vi "Save Data To File.vi"(0 "VISA resource name":refnum<visa-resource-name>, 1 "Memory Waveform Source (0: Channel 1)":i32(ring) items=["Channel 1", "Channel 2", "Channel 3", "Channel 4", "Math", "Memory Waveform 1", "Memory Waveform 2"], 2 "Internal Location (0)":dbl, 5 "File Type (0: Agilent Logic Binary)":i32(ring) items=["Agilent Logic Binary", "ASCII XY ", "CSV", "Binary", "Reference Waveform", "Setup", "Lister", "Masker", "Arbitrary", "Power"], 7 "Waveform Length (2000 points)":i32=2000, 9 "Segment Select (0: All)":i32(ring) items=["All", "Current"], 11 "error in (no error)":errorcluster, 12 "File Name":string, 13 "Enable Max Waveform Length (F: Disable)":bool) -> (4 "VISA resource name out":refnum<visa-resource-name>, 15 "error out":errorcluster)   [LabVIEW 2023, in "Keysight-DSQx3014T.lvlib"]
doc: "Configure the save waveform to file operation."
uses:
  Keysight-DSQx3014T.lvlib
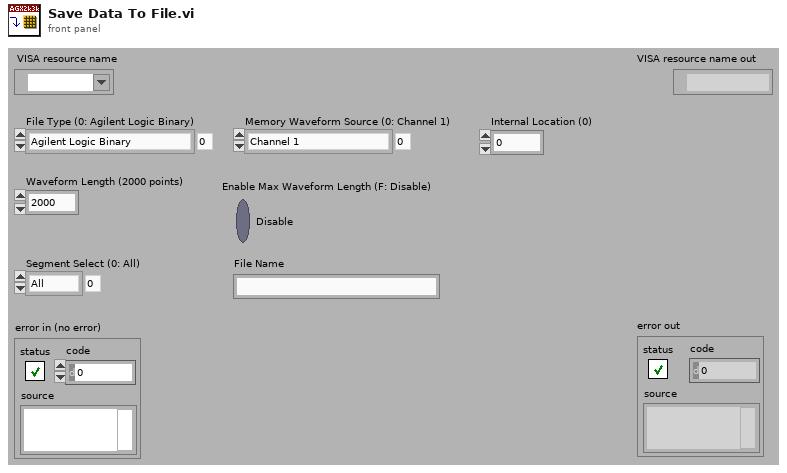
[diagram p1: front panel]
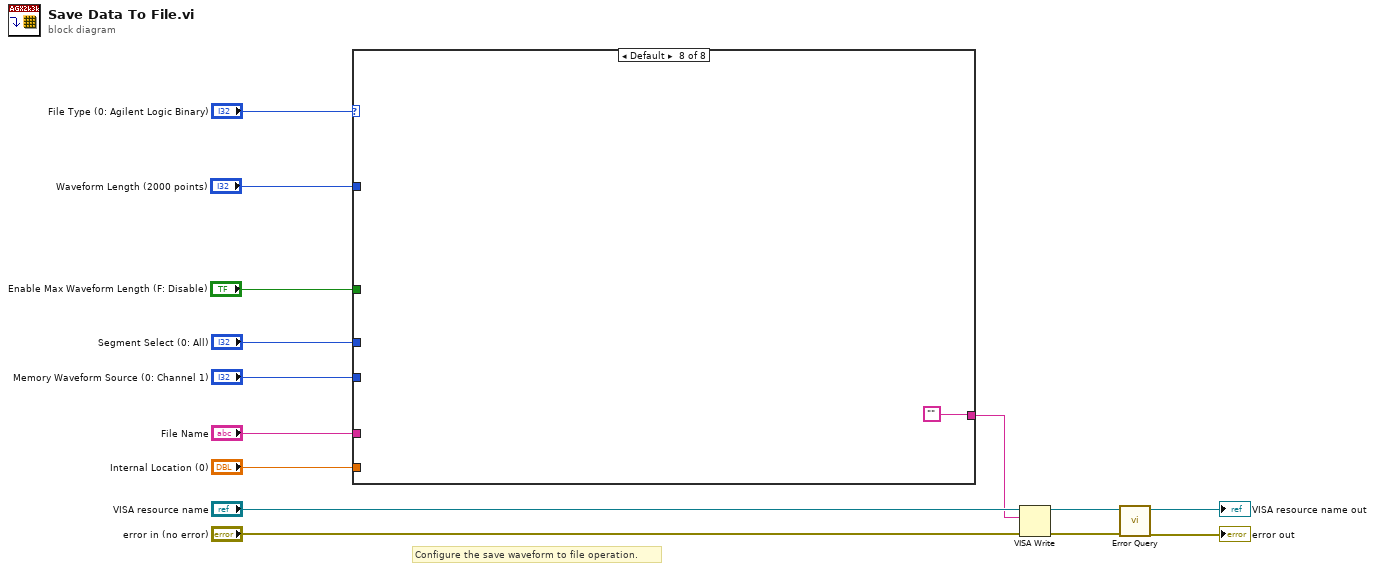
[diagram p0: block diagram]
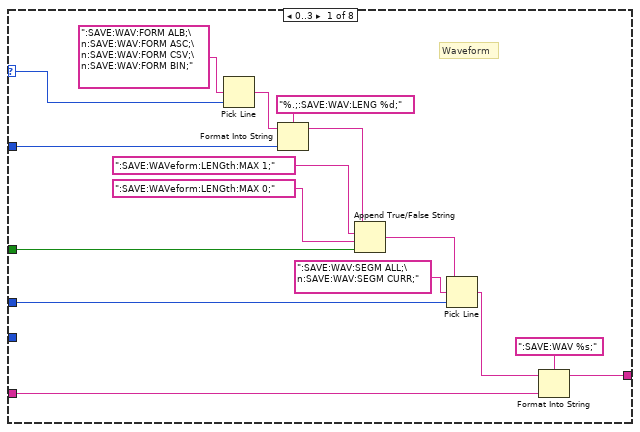
[diagram p2: hidden frame]
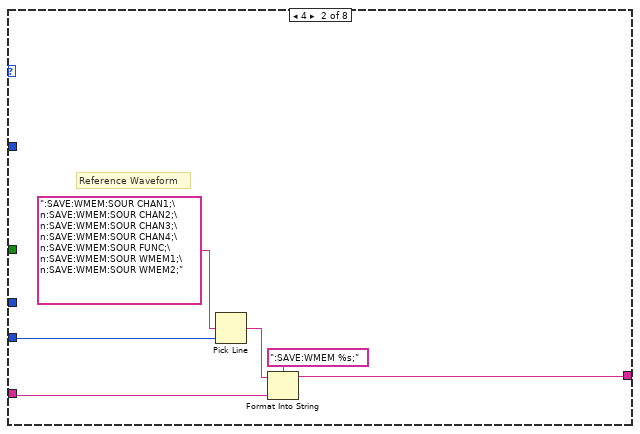
[diagram p3: hidden frame]
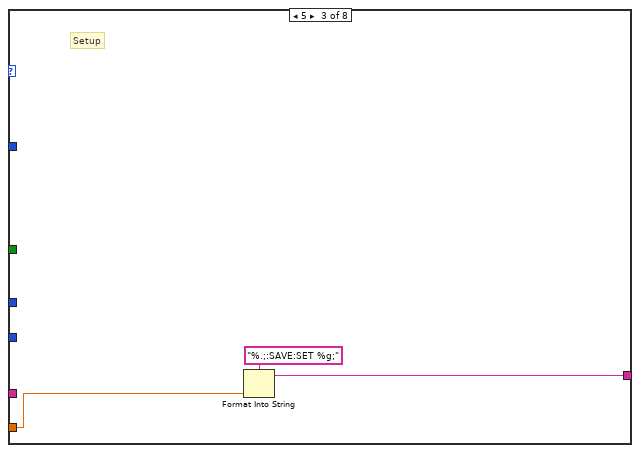
[diagram p4: hidden frame]
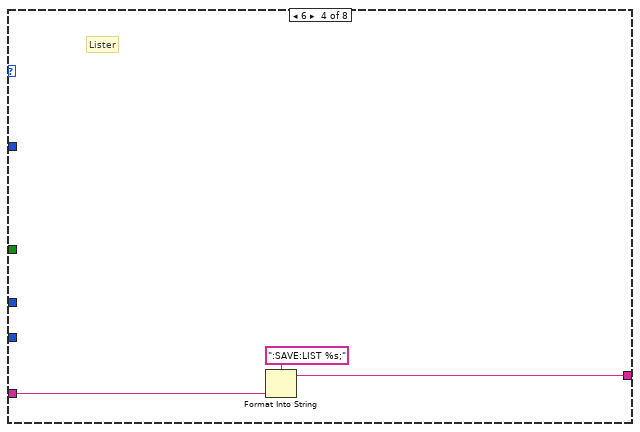
[diagram p5: hidden frame]
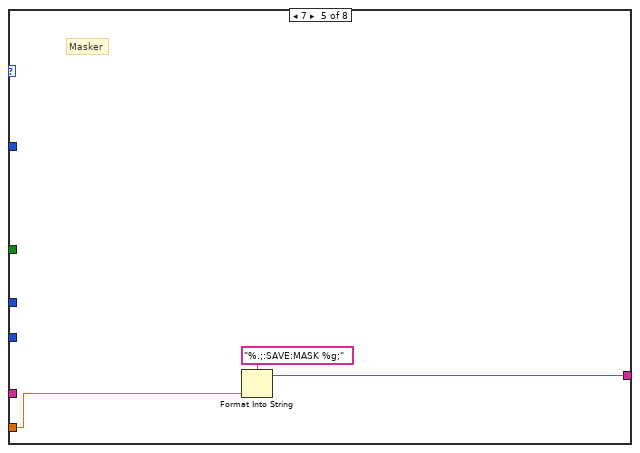
[diagram p6: hidden frame]
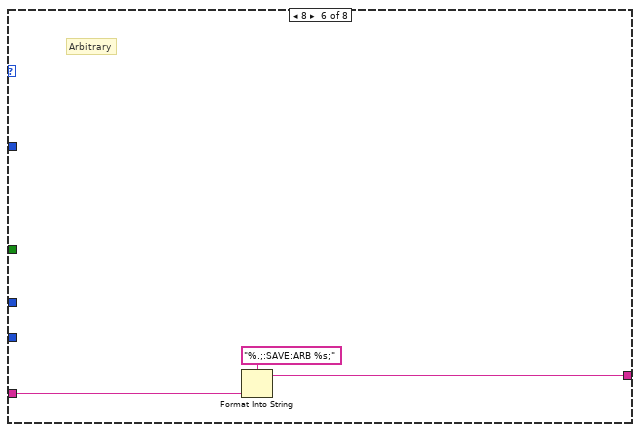
[diagram p7: hidden frame]
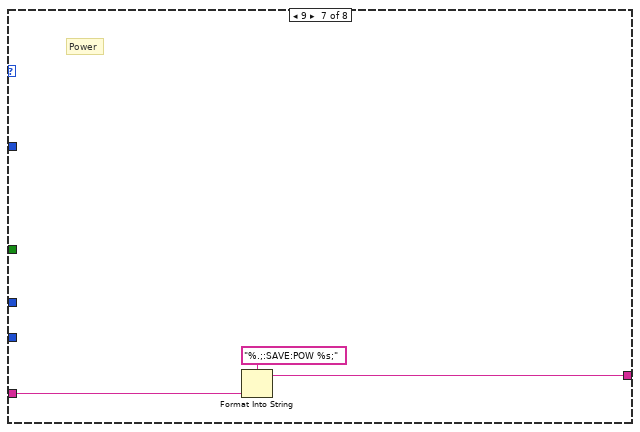
[diagram p8: hidden frame]
diagram:
  # "Configure the save waveform to file operation."
  n1 = case shown="Default" "File Type (0: Agilent Logic Binary)" {
    selector: "File Type (0: Agilent Logic Binary)" -> [w29 _ _ _ _ _ _ _]
    tunnel: "Waveform Length (2000 points)" -> [w26 _ _ _ _ _ _ _]
    tunnel: "Segment Select (0: All)" -> [w25 _ _ _ _ _ _ _]
    tunnel: "File Name" -> [w23 w35 _ w41 _ w46 w49 _]
    tunnel: "Memory Waveform Source (0: Channel 1)" -> [_ w36 _ _ _ _ _ _]
    tunnel: "Internal Location (0)" -> [_ _ w38 _ w44 _ _ _]
    tunnel: [w21 w31 w37 w40 w43 w47 w50 ""] -> w2
    tunnel: "Enable Max Waveform Length (F: Disable)" -> [w19 _ _ _ _ _ _ _]
    frame 0..3 {
      # "Waveform"
      n2 = Pick Line(multi-line string=":SAVE:WAV:FORM ALB;\n:SAVE:WAV:FORM ASC;\n:SAVE:WAV:FORM CSV;\n:SAVE:WAV:FORM BIN;", line index=w29) -> (output string=w27:string)  [unwired: 1 out]
      n3 = Format Into String(format string="%.;:SAVE:WAV:LENG %d;", initial string=w27, w26) -> (resulting string=w16:string)  [unwired: 1 in, 1 out]
      n4 = Append True/False String(1:w19, 2:":SAVE:WAVeform:LENGth:MAX 0;", 3:":SAVE:WAVeform:LENGth:MAX 1;", 4:w16) -> (0:w15:string)
      n5 = Pick Line(string ("")=w15, multi-line string=":SAVE:WAV:SEGM ALL;\n:SAVE:WAV:SEGM CURR;", line index=w25) -> (output string=w22:string)
      n6 = Format Into String(format string=":SAVE:WAV %s;", initial string=w22, w23) -> (resulting string=w21:string)  [unwired: 1 in, 1 out]
    }
    frame 4 {
      # "Reference Waveform"
      n7 = Pick Line(multi-line string=":SAVE:WMEM:SOUR CHAN1;\n:SAVE:WMEM:SOUR CHAN2;\n:SAVE:WMEM:SOUR CHAN3;\n:SAVE:WMEM:SOUR CHAN4;\n:SAVE:WMEM:SOUR FUNC;\n:SAVE:WMEM:SOUR WMEM1;\n:SAVE:WMEM:SOUR WMEM2;", line index=w36) -> (output string=w33:string)  [unwired: 1 out]
      n8 = Format Into String(format string=":SAVE:WMEM %s;", initial string=w33, w35) -> (resulting string=w31:string)  [unwired: 1 in, 1 out]
    }
    frame 5 {
      # "Setup"
      n9 = Format Into String(format string="%.;:SAVE:SET %g;", w38) -> (resulting string=w37:string)  [unwired: 2 in, 1 out]
    }
    frame 6 {
      # "Lister"
      n10 = Format Into String(format string=":SAVE:LIST %s;", w41) -> (resulting string=w40:string)  [unwired: 2 in, 1 out]
    }
    frame 7 {
      # "Masker"
      n11 = Format Into String(format string="%.;:SAVE:MASK %g;", w44) -> (resulting string=w43:string)  [unwired: 2 in, 1 out]
    }
    frame 8 {
      # "Arbitrary"
      n12 = Format Into String(format string="%.;:SAVE:ARB %s;", w46) -> (resulting string=w47:string)  [unwired: 2 in, 1 out]
    }
    frame 9 {
      # "Power"
      n13 = Format Into String(format string="%.;:SAVE:POW %s;", w49) -> (resulting string=w50:string)  [unwired: 2 in, 1 out]
    }
    frame Default {
    }
  }
  n14 = VISA Write(VISA resource name="VISA resource name", write buffer=w2, error in (no error)="error in (no error)") -> (VISA resource name out=w12:refnum<visa-resource-name>, error out=w11:errorcluster)  [unwired: 1 out]
  n15 = call "Error Query.vi"("error in (no error)"=w11, "VISA resource name"=w12) -> ("error out"=→"error out":errorcluster, "VISA resource name out"=→"VISA resource name out":refnum<visa-resource-name>)  [unwired: 8 out]
